vi "Deadzone.vi"(11 "Numeric 2":dbl) -> (3 "Numeric":dbl)   [LabVIEW 2015]
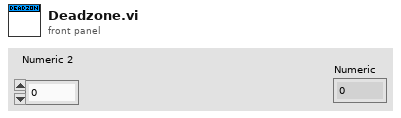
[diagram p1: front panel]
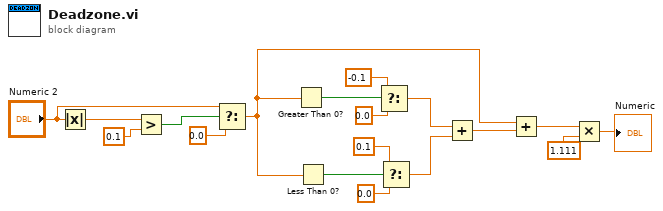
[diagram p0: block diagram]
diagram:
  n1 = Absolute Value(x="Numeric 2") -> (abs(x)=w18:dbl)
  n2 = Greater?(x=w18, y=0.1) -> (0:w16:bool)
  n3 = Select(t="Numeric 2", s=w16, f=0.0) -> (s? t:f=w1:dbl)
  n4 = Greater Than 0?(x=w1) -> (x > 0?=w14:bool)
  n5 = Less Than 0?(x=w1) -> (x < 0?=w13:bool)
  n6 = Select(t=-0.1, s=w14, f=0.0) -> (s? t:f=w8:dbl)
  n7 = Select(t=0.1, s=w13, f=0.0) -> (s? t:f=w7:dbl)
  n8 = Add(x=w8, y=w7) -> (x+y=w6:dbl)
  n9 = Add(x=w1, y=w6) -> (x+y=w4:dbl)
  n10 = Multiply(x=w4, y=1.111) -> (x*y=→"Numeric":dbl)
